vi "Save File General Headers.vi"(7 "LV Program":T1=enum."DOE Stand", 8 "Error In":errorcluster) -> (0 "Error Out":errorcluster, 1 "Debug Log Header":string[](array[string])=["Date", "Time", "Debug Logs"], 2 "Current Header":string[](array[string])=["Date", "Time", "Time (Seconds)", "Current (Amps)", "Voltage (Volts)"], 3 "Summary Header":string[](array[string])=["Date", "Time", "Total Cycle Time (Minutes)", "Cycle Number", "Maximum RPM", "# of Error Codes", "Maximum Current", "IGBT Temperature", "Load Size", "Temperature", "Water Pressure", "Detergent", "Fabric Softener", "Inverter Power (W)", "Raw OOB", "Current Motor Temp (Deg C)"])   [LabVIEW 2016, in "Save File.lvlib"]
uses:
  Save File.lvlib
  File Setup (Public)/Type Definition/Save File DOE LabView Program.ctl
  File Setup.lvlib
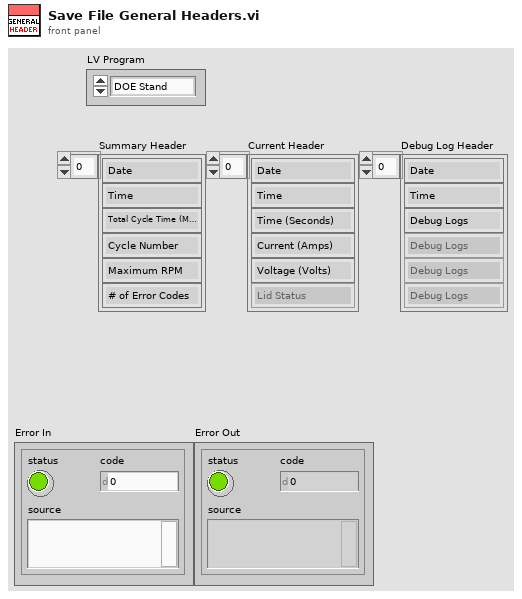
[diagram p1: front panel]
types:
  T1 = typedef "File Setup.lvlib/Save File DOE LabView Program.ctl" = enum16{"No Name Found", "DOE Stand", "Dishwasher Kitchen", "Portable Stand", "HEWH", "Dryer", "Dryer WILT", "HCC", "PRAT", "HEWH RLT", "Refrigeration"}
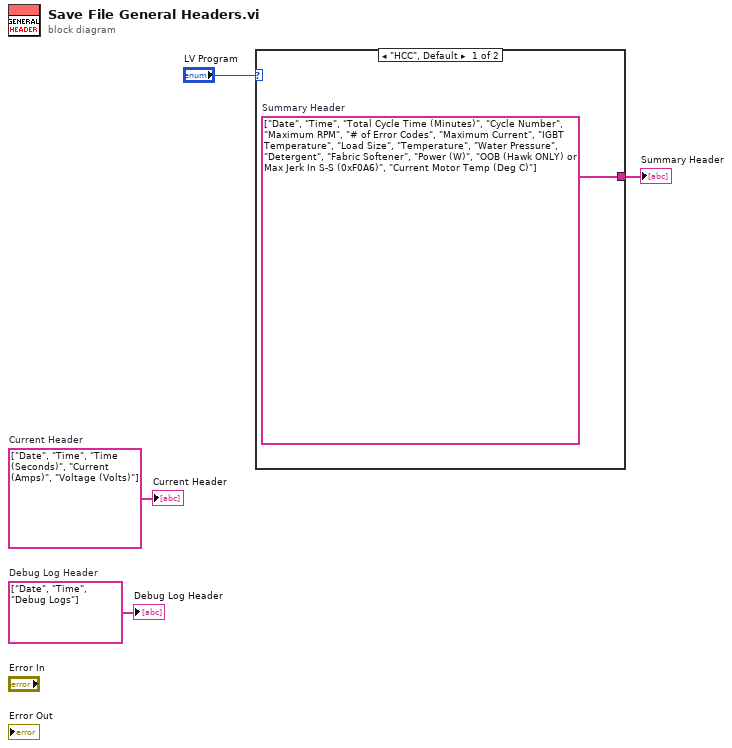
[diagram p0: block diagram]
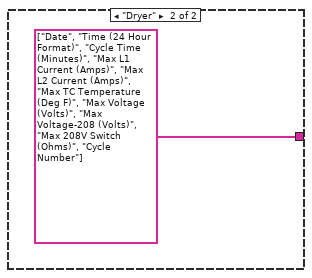
[diagram p2: hidden frame]
diagram:
  w2 = string[] ["Date", "Time", "Debug Logs"]  # Debug Log Header
  w3 = string[] ["Date", "Time", "Time (Seconds)", "Current (Amps)", "Voltage (Volts)"]  # Current Header
  n1 = case shown="\"HCC\", Default" "LV Program" {
    tunnel: [w5 string[] ["Date", "Time (24 Hour Format)", "Cycle Time (Minutes)", "Max L1 Current (Amps)", "Max L2 Current (Amps)", "Max TC Temperature (Deg F)", "Max Voltage (Volts)", "Max Voltage-208 (Volts)", "Max 208V Switch (Ohms)", "Cycle Number"]] -> w4
    frame "HCC", Default {
      w5 = string[] ["Date", "Time", "Total Cycle Time (Minutes)", "Cycle Number", "Maximum RPM", "# of Error Codes", "Maximum Current", "IGBT Temperature", "Load Size", "Temperature", "Water Pressure", "Detergent", "Fabric Softener", "Power (W)", "OOB (Hawk ONLY) or Max Jerk In S-S (0xF0A6)", "Current Motor Temp (Deg C)"]  # Summary Header
    }
    frame "Dryer" {
    }
  }
  "Summary Header" <- w4
  "Current Header" <- w3
  "Debug Log Header" <- w2
